vi "CI_WarningCriticalRangeWrite.vi"(4 "error in (no error)":errorcluster, 5 "Value":u8, 6 "Container State":T2, 7 "Display State In":T1={"StandardColor"=6881066, "WarningColor"=16766208, "CriticalColor"=15671808, "Standard<>Warning Range"=75, "Warning<>Critical Range"=95}) -> (0 "error out":errorcluster, 3 "Display State Out":T1={"StandardColor"=6881066, "WarningColor"=16766208, "CriticalColor"=15671808, "Standard<>Warning Range"=75, "Warning<>Critical Range"=95})   [LabVIEW 2010, in "CapacityIndicator.xctl"]
uses:
  CapacityIndicator.xctl
  <vilib>/_xctls/Container State.ctl
  CI_State.ctl
  <vilib>/_xctls/XControlSupport.lvlib
panel:
  # "Replace the Value Control below with a Control of desired type.\nDo not remove this Control or the others from the connector pane.\nDo not change the connector pane pattern.\nThe Value control should always be the third terminal from top on the input side in the connector pane."
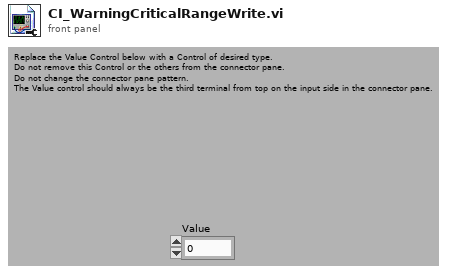
[diagram p1: front panel]
types:
  T1 = typedef "CapacityIndicator.xctl/CI_State.ctl" = cluster{"StandardColor":u32, "WarningColor":u32, "CriticalColor":u32, "Standard<>Warning Range":u8, "Warning<>Critical Range":u8}
  T2 = typedef "XControlSupport.lvlib/Container State.ctl" = cluster{"Indicator?":bool, "Run Mode?":bool, " Refnum":refnum<vi>}
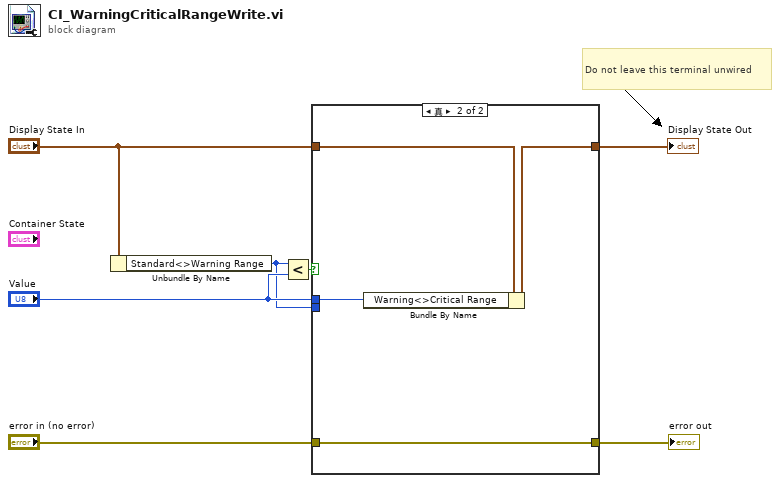
[diagram p0: block diagram]
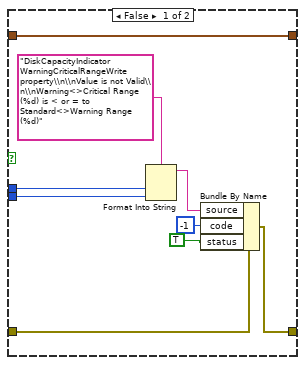
[diagram p2: hidden frame]
diagram:
  # "Do not leave this terminal unwired"
  n1 = Unbundle By Name("Display State In") -> ("Standard<>Warning Range"=w1:u8)
  n2 = Less?(x=w1, y="Value") -> (x < y?=w7:bool)
  n3 = case shown="真" w7 {
    tunnel: "Display State In" -> [w16 w20]
    tunnel: [w16 w19] -> w5
    tunnel: "Value" -> [w15 w18]
    tunnel: [w11 w17] -> w3
    tunnel: "error in (no error)" -> [w12 w17]
    tunnel: w1 -> [w14 _]
    frame False {
      n4 = Format Into String(format string="DiskCapacityIndicator WarningCriticalRangeWrite property\\n\\nValue is not Valid\\n\\nWarning<>Critical Range (%d) is < or = to Standard<>Warning Range (%d)", w15, w14) -> (resulting string=w9:string)  [unwired: 2 in, 1 out]
      n5 = Bundle By Name(cluster=w12, "source"=w9, "code"=-1, "status"=TRUE) -> (w11:errorcluster)
    }
    frame True {
      n6 = Bundle By Name(cluster=w20, "Warning<>Critical Range"=w18) -> (w19:T1)
    }
  }
  "error out" <- w3
  "Display State Out" <- w5
